vi "Close Subscription Policy.vi"(8 "error in (no error)":errorcluster, 11 "Subscription Policy Reference":T1) -> (0 "error out (Unsubscribe?)":errorcluster)   [LabVIEW 2020, in "MVA Framework.lvlib" / "IMediator.lvlib" / "ISubscriptionPolicy.lvclass"]
doc: "关闭订阅策略"
uses:
  ISubscriptionPolicy.lvclass
  ISubscriptionPolicy Reference.ctl
  ISubscriptionPolicy.lvclass/ISubscriptionPolicy.ctl
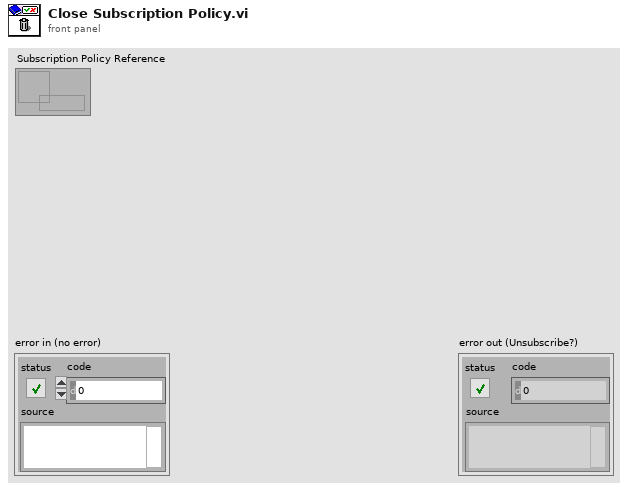
[diagram p1: front panel]
types:
  T1 = typedef "MVA Framework.lvlib/IMediator.lvlib/ISubscriptionPolicy.lvclass/ISubscriptionPolicy Reference.ctl" = refnum<data-value>
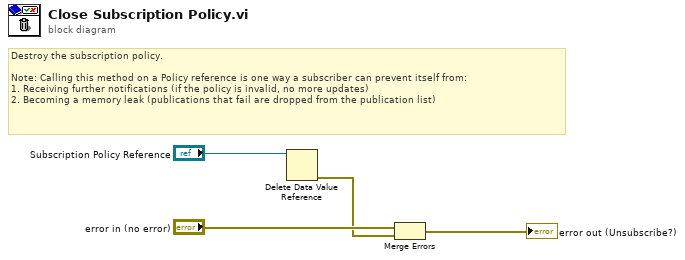
[diagram p0: block diagram]
diagram:
  # "Destroy the subscription policy.\n\nNote: Calling this method on a Policy reference is one way a subscriber can prevent itself from:\n1. Receiving further notifications (if the policy is invalid, no more updates)\n2. Becoming a memory leak (publications that fail are dropped from the publication list)"
  n1 = Delete Data Value Reference(data value reference="Subscription Policy Reference") -> (error out=w1:errorcluster)  [unwired: 1 in, 1 out]
  n2 = Merge Errors("error in (no error)", w1) -> (→"error out (Unsubscribe?)":errorcluster)
